vi "master.vi"   [LabVIEW 2016]
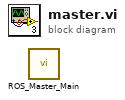
[diagram p0: block diagram]
diagram:
  n1 = call <userlib>:"ROS_Master_Main.vi"() -> ()  [unwired: 4 in]
